vi "insert_edge_nodes.vi"(9 "destination-node":refnum<class "Node.lvclass">, 10 "source-node":refnum<class "Node.lvclass">, 11 "digraph":refnum<class "DiGraph.lvclass">) -> (1 "edge unchanged?":bool, 2 "edge already included?":bool, 3 "digraph out":refnum<class "DiGraph.lvclass">)   [LabVIEW 2020]
uses:
  DiGraph.lvclass
  Node/Node.lvclass
  Edge/Edge.lvclass
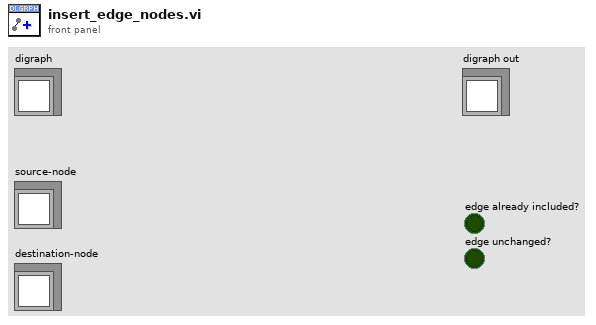
[diagram p1: front panel]
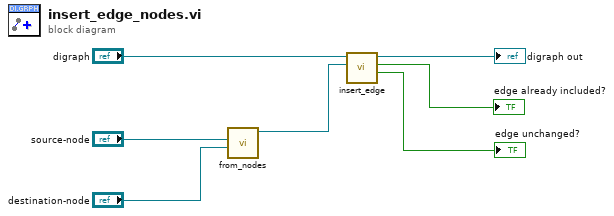
[diagram p0: block diagram]
diagram:
  n1 = call "from_nodes.vi"("destination-node"="destination-node", "source-node"="source-node") -> ("new edge"=w2:refnum<class "Edge.lvclass">)  [unwired: 9 in]
  n2 = call-dynamic "insert_edge.vi"("edge"=w2, "digraph"="digraph") -> ("edge unchanged?"=→"edge unchanged?":bool, "edge already included?"=→"edge already included?":bool, "digraph out"=→"digraph out":refnum<class "DiGraph.lvclass">)  [unwired: 7 in]
